vi "Create RDB Cluster.vi"(8 "error out":errorcluster, 11 "Channel Refs":T4[](array[typedef]) format="%.0x") -> (0 "error out 2":errorcluster, 3 "Array":T1)   [LabVIEW 2018, in "Vires VTD System Explorer.lvlib"]
uses:
  Vires VTD System Explorer.lvlib
  <vilib>/NI Veristand/Custom Device API/Custom Device Item Ref.ctl
  RDB Data.ctl
  RDB/RDB Object.ctl
  RDB/RDB Player Object.ctl
  <vilib>/NI Veristand/Custom Device API/Get Item Property (Variant).vi
  RDB/RDB.lvlib
  <vilib>/NI Veristand/Custom Device API/Custom Device API.lvlib
  Shared/Vires VTD Shared.lvlib
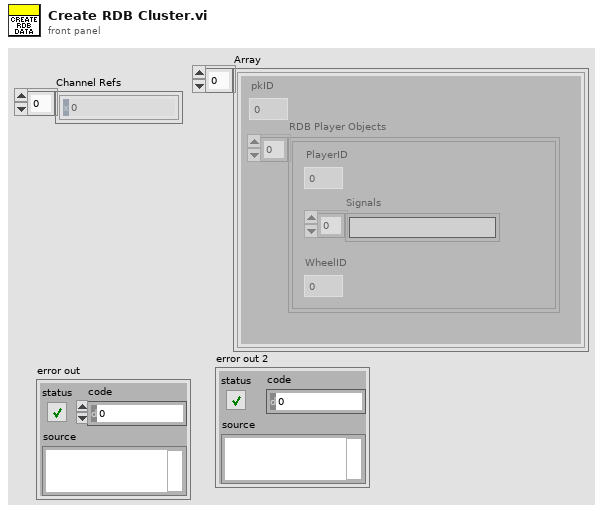
[diagram p1: front panel]
types:
  T1 = typedef "Vires VTD Shared.lvlib/RDB Data.ctl" = T2[]
  T2 = typedef "RDB.lvlib/RDB Object.ctl" = cluster{"pkID":i32, "RDB Player Objects":T3[]}
  T3 = typedef "RDB.lvlib/RDB Player Object.ctl" = cluster{"PlayerID":i32, "Signals":string[], "WheelID":i32}
  T4 = typedef "Custom Device API.lvlib/Custom Device Item Ref.ctl" = u64
  T5 = enum16{"open", "replace", "create", "open or create", "replace or create", "replace or create with confirmation"}
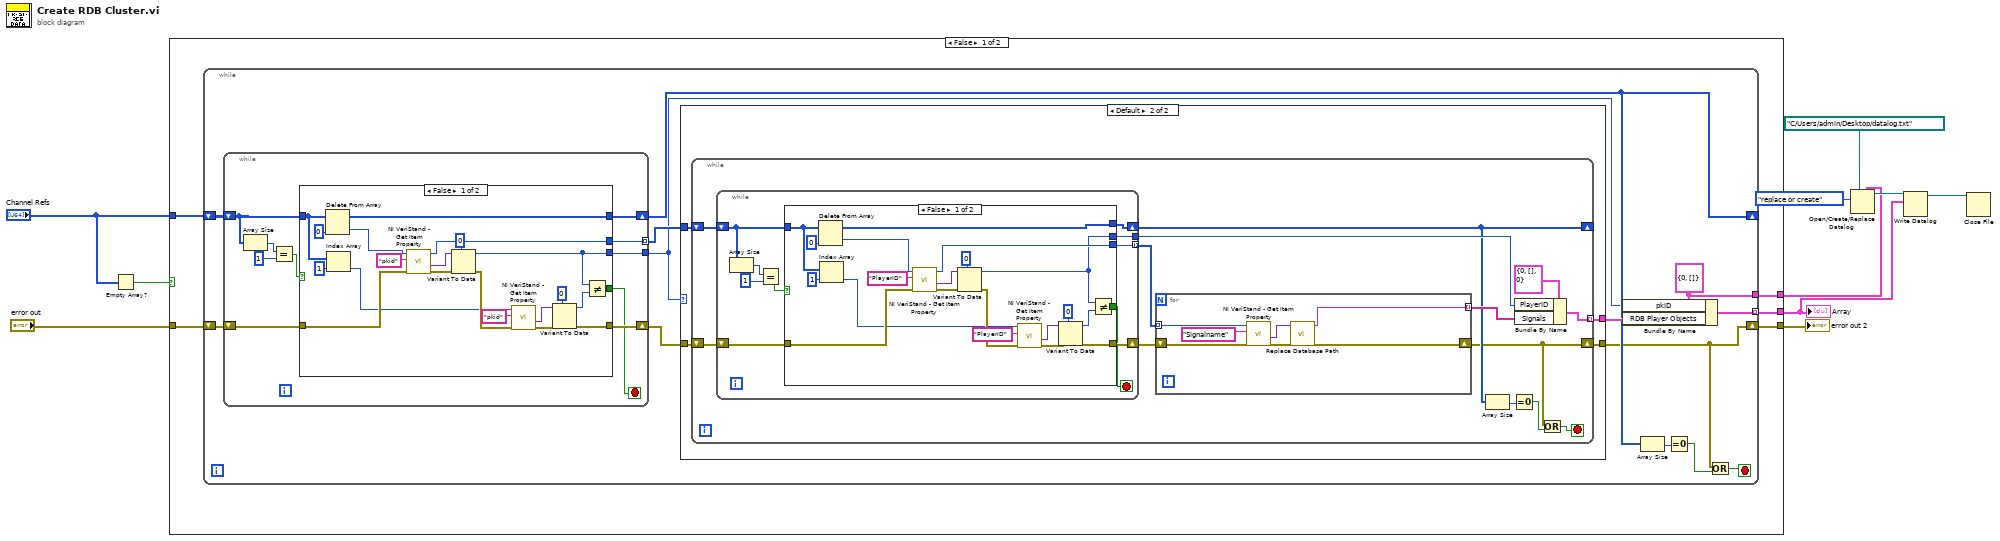
[diagram p0: block diagram]
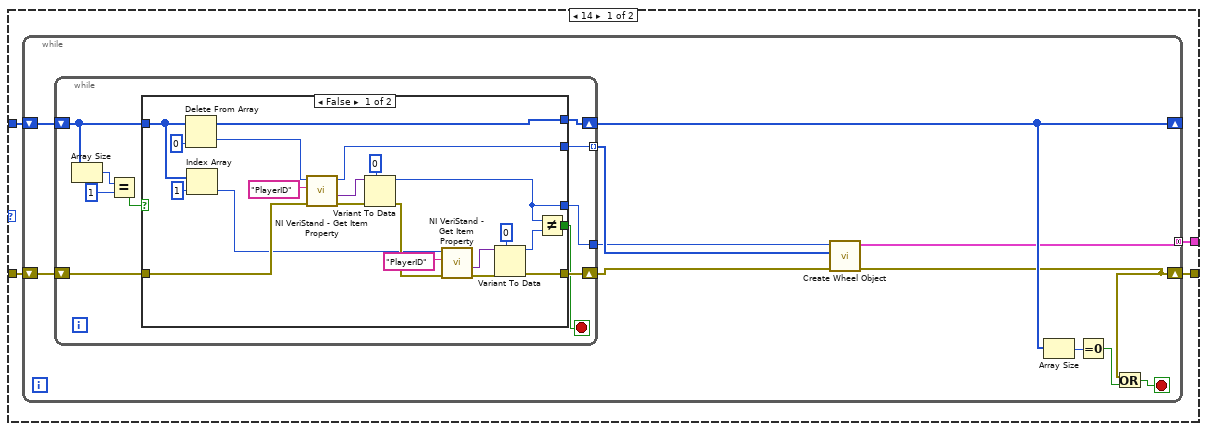
[diagram p2: hidden frame]
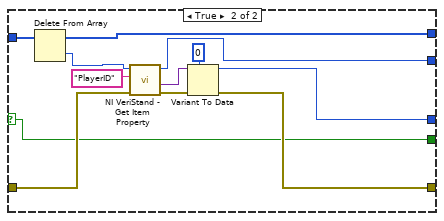
[diagram p3: hidden frame]
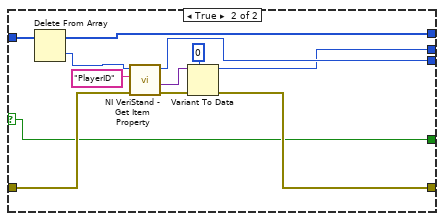
[diagram p4: hidden frame]
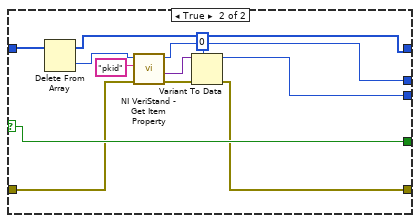
[diagram p5: hidden frame]
diagram:
  n1 = Empty Array?(array="Channel Refs") -> (empty?=w7:bool)
  n2 = case shown="False" w7 {
    tunnel: "Channel Refs" -> [w15 _]
    tunnel: "error out" -> [w14 w197]
    tunnel: [w13 w197] -> w9
    tunnel: [w12 _] -> w1
    tunnel: [w11 _] -> w3
    frame False {
      n3 = while {
        shift-right: [w20] -> _
        shift-left: w15 -> [w28]
        shift-right: [w19] -> w13
        shift-left: w14 -> [w24]
        tunnel: [w18] -> w12 mode=indexing
        tunnel: [w16] -> w11
        stop <- w21 stop-if-true
        w16 = T2 {"pkID"=0, "RDB Player Objects"=[]} ("RDB Object")
        n4 = while {
          shift-right: [w163] -> w27
          shift-left: w24 -> [w162]
          tunnel: [w160] -> w26 mode=indexing
          tunnel: [w159] -> w17
          shift-right: [w158] -> w20
          shift-left: w28 -> [w157]
          stop <- w161 stop-if-true
          n5 = Array Size(array=w157) -> (size(s)=w156:i32)
          n6 = Equal?(x=w156, y=1) -> (x = y?=w154:bool)
          n7 = case shown="False" w154 {
            selector: w154 -> [_ w196]
            tunnel: [w177 w189] -> w163
            tunnel: w162 -> [w176 w190]
            tunnel: [w172 w196] -> w161
            tunnel: [w171 w187] -> w160
            tunnel: [w170 w188] -> w159
            tunnel: [w166 w185] -> w158
            tunnel: w157 -> [w164 w186]
            frame False {
              n8 = Delete From Array(array=w164, index=0) -> (deleted portion=w167:T4, array with subset deleted=w166:T4[])  [unwired: 1 in]
              n9 = Index Array(array=w164, index=1) -> (element=w165:T4)
              n10 = call-poly <vilib>:"NI VeriStand - Get Item Property.vi"("error in (no error)"=w176, "Property Name"="pkid", "Item Ref in"=w167) -> ("error out"=w182:errorcluster, "Value"=w181:variant, "Item Ref out"=w171:T4)  [unwired: 5 in, 1 out]
              n11 = Variant To Data(error in=w182, type=u8 0, Variant=w181) -> (data=w170:u8, error out=w180:errorcluster)
              n12 = call-poly <vilib>:"NI VeriStand - Get Item Property.vi"("error in (no error)"=w180, "Property Name"="pkid", "Item Ref in"=w165) -> ("error out"=w179:errorcluster, "Value"=w178:variant)  [unwired: 5 in, 2 out]
              n13 = Variant To Data(error in=w179, type=u8 0, Variant=w178) -> (data=w174:u8, error out=w177:errorcluster)
              n14 = Not Equal?(x=w170, y=w174) -> (x != y?=w172:bool)
            }
            frame True {
              n15 = Delete From Array(array=w186) -> (deleted portion=w191:T4, array with subset deleted=w185:T4[])  [unwired: 2 in]
              n16 = call-poly <vilib>:"NI VeriStand - Get Item Property.vi"("error in (no error)"=w190, "Property Name"="pkid", "Item Ref in"=w191) -> ("error out"=w194:errorcluster, "Value"=w193:variant, "Item Ref out"=w187:T4)  [unwired: 5 in, 1 out]
              n17 = Variant To Data(error in=w194, type=u8 0, Variant=w193) -> (data=w188:u8, error out=w189:errorcluster)
            }
          }
        }
        n18 = case shown="Default" w17 {
          tunnel: w27 -> [w31 w90]
          tunnel: w26 -> [w32 w89]
          tunnel: [w30 w88] -> w25
          tunnel: [w29 w87] -> w19
          frame 14 {
            n19 = while {
              shift-right: [w38] -> _
              shift-left: w32 -> [w42]
              shift-right: [w34] -> w29
              shift-left: w31 -> [w43]
              tunnel: [w33] -> w30 mode=concatenating
              stop <- w37 stop-if-true
              n20 = while {
                shift-right: [w53] -> w40
                shift-left: w43 -> [w52]
                tunnel: [w50] -> w41 mode=indexing
                tunnel: [w49] -> w39
                shift-right: [w44] -> w38
                shift-left: w42 -> [w46]
                stop <- w51 stop-if-true
                n21 = Array Size(array=w46) -> (size(s)=w47:i32)
                n22 = Equal?(x=w47, y=1) -> (x = y?=w45:bool)
                n23 = case shown="False" w45 {
                  selector: w45 -> [_ w80]
                  tunnel: [w67 w81] -> w53
                  tunnel: w52 -> [w66 w82]
                  tunnel: [w62 w80] -> w51
                  tunnel: [w61 w79] -> w50
                  tunnel: [w60 w78] -> w49
                  tunnel: w46 -> [w59 w77]
                  tunnel: [w54 w76] -> w44
                  frame False {
                    n24 = Delete From Array(array=w59, index=0) -> (deleted portion=w55:T4, array with subset deleted=w54:T4[])  [unwired: 1 in]
                    n25 = Index Array(array=w59, index=1) -> (element=w58:T4)
                    n26 = call-poly <vilib>:"NI VeriStand - Get Item Property.vi"("error in (no error)"=w66, "Property Name"="PlayerID", "Item Ref in"=w55) -> ("error out"=w72:errorcluster, "Value"=w71:variant, "Item Ref out"=w61:T4)  [unwired: 5 in, 1 out]
                    n27 = Variant To Data(error in=w72, type=u8 0, Variant=w71) -> (data=w60:u8, error out=w70:errorcluster)
                    n28 = call-poly <vilib>:"NI VeriStand - Get Item Property.vi"("error in (no error)"=w70, "Property Name"="PlayerID", "Item Ref in"=w58) -> ("error out"=w69:errorcluster, "Value"=w68:variant)  [unwired: 5 in, 2 out]
                    n29 = Variant To Data(error in=w69, type=u8 0, Variant=w68) -> (data=w64:u8, error out=w67:errorcluster)
                    n30 = Not Equal?(x=w60, y=w64) -> (x != y?=w62:bool)
                  }
                  frame True {
                    n31 = Delete From Array(array=w77) -> (deleted portion=w75:T4, array with subset deleted=w76:T4[])  [unwired: 2 in]
                    n32 = call-poly <vilib>:"NI VeriStand - Get Item Property.vi"("error in (no error)"=w82, "Property Name"="PlayerID", "Item Ref in"=w75) -> ("error out"=w84:errorcluster, "Value"=w85:variant, "Item Ref out"=w79:T4)  [unwired: 5 in, 1 out]
                    n33 = Variant To Data(error in=w84, type=u8 0, Variant=w85) -> (data=w78:u8, error out=w81:errorcluster)
                  }
                }
              }
              n34 = call "Create Wheel Object.vi"("error out 2"=w40, "Array"=w41, "Numeric"=w39) -> ("error out"=w34:errorcluster, "Array 2"=w33:T3[])  [unwired: 7 in]
              n35 = Array Size(array=w38) -> (size(s)=w36:i32)
              n36 = Equal To 0?(x=w36) -> (x = 0?=w35:bool)
              n37 = Or(x=w34, y=w35) -> (x .or. y?=w37:bool)
            }
          }
          frame Default {
            n38 = while {
              shift-right: [w96] -> _
              shift-left: w89 -> [w102]
              shift-right: [w92] -> w87
              shift-left: w90 -> [w103]
              tunnel: [w91] -> w88 mode=indexing
              stop <- w95 stop-if-true
              n39 = while {
                shift-right: [w113] -> w100
                shift-left: w103 -> [w112]
                tunnel: [w110] -> w101 mode=indexing
                tunnel: [w109] -> w98
                shift-right: [w104] -> w96
                shift-left: w102 -> [w106]
                stop <- w111 stop-if-true
                n40 = Array Size(array=w106) -> (size(s)=w107:i32)
                n41 = Equal?(x=w107, y=1) -> (x = y?=w105:bool)
                n42 = case shown="False" w105 {
                  selector: w105 -> [_ w140]
                  tunnel: [w127 w141] -> w113
                  tunnel: w112 -> [w126 w142]
                  tunnel: [w122 w140] -> w111
                  tunnel: [w121 w139] -> w110
                  tunnel: [w120 w138] -> w109
                  tunnel: w106 -> [w119 w137]
                  tunnel: [w114 w136] -> w104
                  frame False {
                    n43 = Delete From Array(array=w119, index=0) -> (deleted portion=w115:T4, array with subset deleted=w114:T4[])  [unwired: 1 in]
                    n44 = Index Array(array=w119, index=1) -> (element=w118:T4)
                    n45 = call-poly <vilib>:"NI VeriStand - Get Item Property.vi"("error in (no error)"=w126, "Property Name"="PlayerID", "Item Ref in"=w115) -> ("error out"=w132:errorcluster, "Value"=w131:variant, "Item Ref out"=w121:T4)  [unwired: 5 in, 1 out]
                    n46 = Variant To Data(error in=w132, type=u8 0, Variant=w131) -> (data=w120:u8, error out=w130:errorcluster)
                    n47 = call-poly <vilib>:"NI VeriStand - Get Item Property.vi"("error in (no error)"=w130, "Property Name"="PlayerID", "Item Ref in"=w118) -> ("error out"=w129:errorcluster, "Value"=w128:variant)  [unwired: 5 in, 2 out]
                    n48 = Variant To Data(error in=w129, type=u8 0, Variant=w128) -> (data=w124:u8, error out=w127:errorcluster)
                    n49 = Not Equal?(x=w120, y=w124) -> (x != y?=w122:bool)
                  }
                  frame True {
                    n50 = Delete From Array(array=w137) -> (deleted portion=w135:T4, array with subset deleted=w136:T4[])  [unwired: 2 in]
                    n51 = call-poly <vilib>:"NI VeriStand - Get Item Property.vi"("error in (no error)"=w142, "Property Name"="PlayerID", "Item Ref in"=w135) -> ("error out"=w144:errorcluster, "Value"=w145:variant, "Item Ref out"=w139:T4)  [unwired: 5 in, 1 out]
                    n52 = Variant To Data(error in=w144, type=u8 0, Variant=w145) -> (data=w138:u8, error out=w141:errorcluster)
                  }
                }
              }
              n53 = for {
                tunnel: w101 -> [w149] mode=indexing
                shift-right: [w147] -> w92
                shift-left: w100 -> [w150]
                tunnel: [w148] -> w99 mode=indexing
                n54 = call-poly <vilib>:"NI VeriStand - Get Item Property.vi"("error in (no error)"=w150, "Property Name"="Signalname", "Item Ref in"=w149) -> ("error out"=w152:errorcluster, "Value"=w153:variant)  [unwired: 5 in, 2 out]
                n55 = call "Replace Database Path.vi"("error in (no error)"=w152, "Value"=w153) -> ("error out"=w147:errorcluster, "Property Name"=w148:string)  [unwired: 8 in]
              }
              n56 = Array Size(array=w96) -> (size(s)=w94:i32)
              n57 = Equal To 0?(x=w94) -> (x = 0?=w93:bool)
              n58 = Bundle By Name(cluster=T3 {"PlayerID"=0, "Signals"=[], "WheelID"=0} ("RDB Player Objects"), "PlayerID"=w98, "Signals"=w99) -> (w91:T3)
              n59 = Or(x=w92, y=w93) -> (x .or. y?=w95:bool)
            }
          }
        }
        n60 = Bundle By Name(cluster=w16, "pkID"=w17, "RDB Player Objects"=w25) -> (w18:T2)
        n61 = Array Size(array=w20) -> (size(s)=w22:i32)
        n62 = Equal To 0?(x=w22) -> (x = 0?=w23:bool)
        n63 = Or(x=w19, y=w23) -> (x .or. y?=w21:bool)
      }
    }
    frame True {
    }
  }
  "Array" <- w1
  "error out 2" <- w9
  n64 = Open/Create/Replace Datalog(5:w3, 10:T5."replace or create" ("operation (0:open)"), 11:path "C:/Users/admin/Desktop/datalog.txt" ("datalog path (use dialog)")) -> (3:w4:refnum<k1>)  [unwired: 3 in, 2 out]
  n65 = Write Datalog(6:w1, 7:w4) -> (3:w2:refnum<k1>)  [unwired: 1 in, 1 out]
  n66 = Close File(refnum=w2) -> ()  [unwired: 1 in, 2 out]
